vi "Poisson Randomize Array.vi"(11 "Array":dbl[](array[numeric])) -> (3 "Poisson Randomized Array":dbl[](array[numeric]))   [LabVIEW 2021, in "Arrays.lvlib"]
uses:
  Arrays.lvlib
  ab975498-e198-4d48-a299-ae221b9a83d4.vi
  ab975498-e198-4d48-a299-ae221b9a83d4.vi/539bd7ec-d9e8-460f-a56d-a449b4a86a5e.vi
  Error/Error.lvlib
  Math/Math.lvlib
panel:
  out "Error Out":errorcluster
  in  "Error In":errorcluster
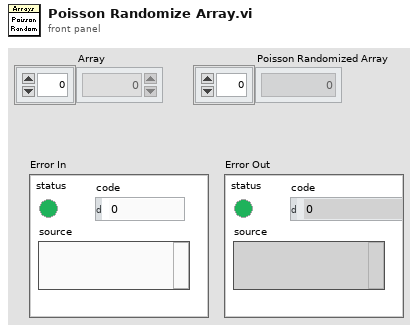
[diagram p1: front panel]
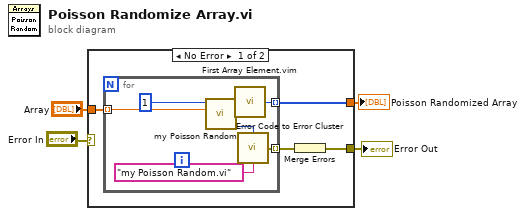
[diagram p0: block diagram]
diagram:
  n1 = case shown="No Error" "Error In" {
    selector: "Error In" -> [_ w17]
    tunnel: [w8 w16] -> w4
    tunnel: "Array" -> [w7 w16]
    tunnel: [w5 w17] -> w1
    frame No Error {
      n2 = for {
        tunnel: w7 -> [w15] mode=indexing
        tunnel: [w12] -> w8 mode=indexing
        tunnel: [w10] -> w6 mode=indexing
        n3 = call "my Poisson Random.vi"("lambda"=w15, "samples (1)"=1 ("samples")) -> ("error"=w11:i32, "Poisson random data"=w13:i32[])  [unwired: 8 in]
        n4 = call "First Array Element.vim"("Array"=w13) -> ("First Element"=w12:i32)  [unwired: 8 in]
        n5 = call "Error Code to Error Cluster.vi"("Error Code"=w11, "Error Source"="my Poisson Random.vi") -> ("Error Out"=w10:errorcluster)  [unwired: 13 in]
      }
      n6 = Merge Errors(w6) -> (w5:errorcluster)
    }
    frame Error {
    }
  }
  "Poisson Randomized Array" <- w4
  "Error Out" <- w1
